vi "Test Selector Dialog.vi"(5 "Directory":path, 6 "Test Program":string, 7 "Test Names":string[](array[string]), 8 "error in":errorcluster, 9 "Test Available":bool[](array[boolean]), 10 "Limited Functional":bool[](array[boolean]), 11 "Test Selector":refnum<class "Test Selector.lvclass">) -> (0 "error out":errorcluster, 1 "Cancelled?":bool, 2 "Selected Tests":bool[](array[boolean]), 3 "Test Selector out":refnum<class "Test Selector.lvclass">, 4 "Limited Functional Flag":bool)   [LabVIEW 2019, in "Test Selector.lvlib" / "Test Selector.lvclass"]
uses:
  Test Selector.lvclass
  Test Selector.lvclass/Test Selector.ctl
  Accessors/Write Limited Functional Flag.vi
  Accessors/Read Limited Functional.vi
  Accessors/Read Selected Tests.vi
  Accessors/Read Test Available.vi
  Accessors/Write LstBox Refnum.vi
  Accessors/Write Test Names.vi
  Accessors/Write Limited Functional.vi
  Accessors/Write Test Available.vi
  Accessors/Write Test Program.vi
  Accessors/Write MissionLogo.vi
  Accessors/Write Directory.vi
  Accessors/Read Limited Functional Flag.vi
  Private/Fill Test Names.vi
  Private/Apply Symbols.vi
  Private/Process Selection.vi
panel:
  in  "Ltd Fnc":bool
  in  "Clear All":bool
  in  "Select All":bool
  in  "CANCEL":bool
  in  "DONE":bool
  in  "Selector":i32[](listbox)
  out "Dialog":string
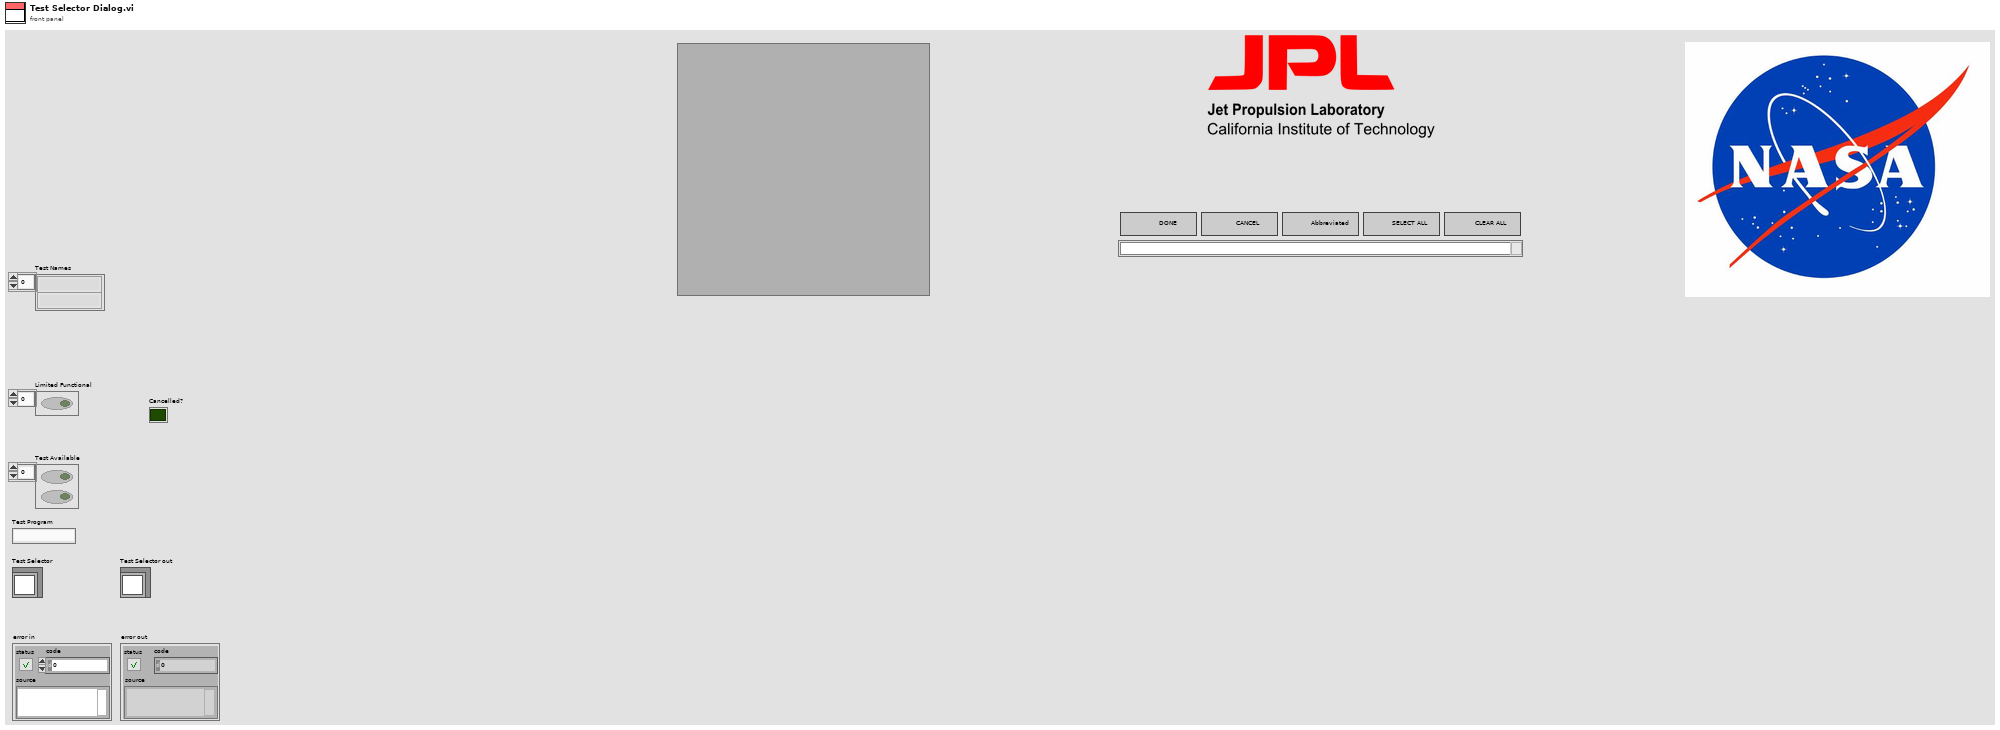
[diagram p1: front panel]
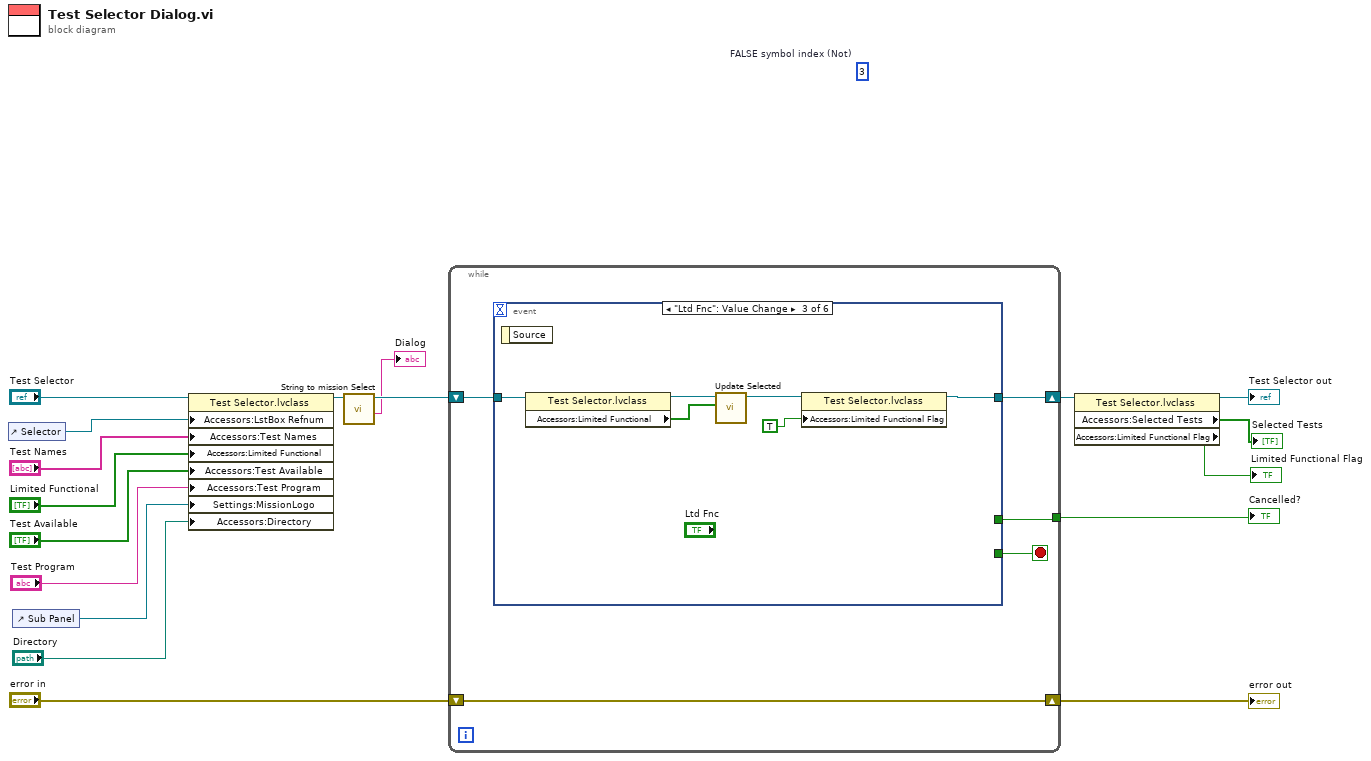
[diagram p0: block diagram]
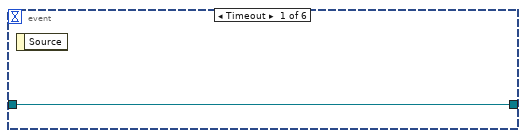
[diagram p2: hidden frame]
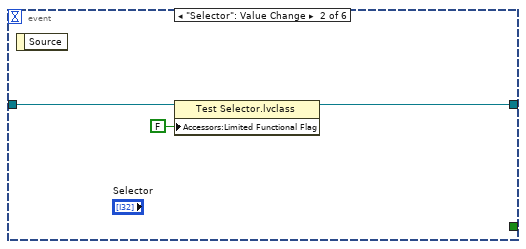
[diagram p3: hidden frame]
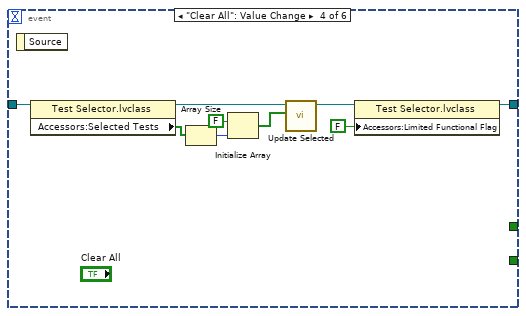
[diagram p4: hidden frame]
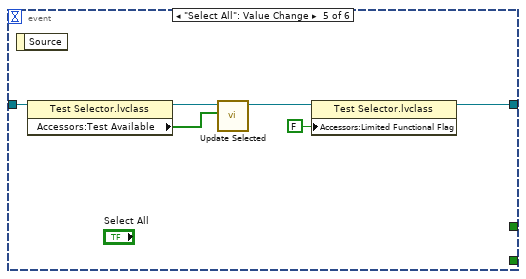
[diagram p5: hidden frame]
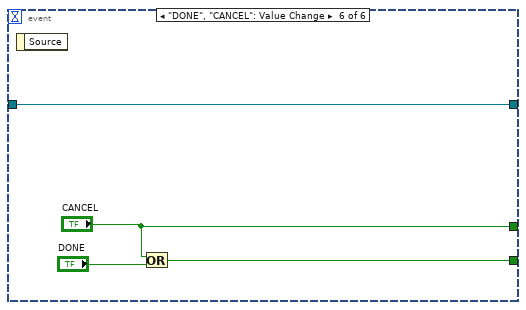
[diagram p6: hidden frame]
diagram:
  (unwired) 3  # FALSE symbol index (Not)
  n1 = control-ref of="Selector"() -> (w15:refnum<vi>)
  n2 = control-ref of="Sub Panel"() -> (w1:refnum<vi>)
  n3 = property class="Test Selector.lvclass"(reference="Test Selector", "Accessors:LstBox Refnum"=w15, "Accessors:Test Names"="Test Names", "Accessors:Limited Functional"="Limited Functional", "Accessors:Test Available"="Test Available", "Accessors:Test Program"="Test Program", "Settings:MissionLogo"=w1, "Accessors:Directory"="Directory") -> (reference out=w10:refnum<class "Test Selector.lvclass">)  [unwired: 1 in, 1 out]
  n4 = call "String to mission Select.vi"("Test Selector in"=w10) -> ("Test Dialog"=→"Dialog":string, "Test Selector out"=w9:refnum<class "Test Selector.lvclass">)  [unwired: 8 in, 1 out]
  n5 = while {
    shift-right: [w23] -> w18
    shift-left: "error in" -> [w23]
    shift-right: [w21] -> w8
    shift-left: w9 -> [w22]
    tunnel: [w19] -> w16
    stop <- w20 stop-if-true
    n6 = event shown="[2] \"Ltd Fnc\": Value Change" {
      selector: _ -> [_ _ _ _ _ _]
      dyn-events: _ -> [_ _ _ _ _ _]
      timeout: _ -> [_ _ _ _ _ _]
      tunnel: w22 -> [w24 w27 w33 w42 w48 w52]
      tunnel: [w24 w26 w29 w35 w44 w52] -> w21
      tunnel: [_ _ _ _ _ w50] -> w20
      tunnel: [_ _ _ _ _ "CANCEL"] -> w19
      event Timeout {
        n7 = event-data() -> ()  [unwired: 1 in, 1 out]
      }
      event "Selector": Value Change {
        n8 = event-data() -> ()  [unwired: 1 in, 1 out]
        n9 = property class="Test Selector.lvclass"(reference=w27, "Accessors:Limited Functional Flag"=FALSE ("Limited Functional Flag")) -> (reference out=w26:refnum<class "Test Selector.lvclass">)  [unwired: 1 in, 1 out]
      }
      event "Ltd Fnc": Value Change {
        n10 = event-data() -> ()  [unwired: 1 in, 1 out]
        n11 = property class="Test Selector.lvclass"(reference=w33) -> (reference out=w32:refnum<class "Test Selector.lvclass">, "Accessors:Limited Functional"=w31:bool[])  [unwired: 1 in, 1 out]
        n12 = call "Update Selected.vi"("Array"=w31, "Test Selector in"=w32) -> ("Test Selector out"=w30:refnum<class "Test Selector.lvclass">)  [unwired: 8 in, 1 out]
        n13 = property class="Test Selector.lvclass"(reference=w30, "Accessors:Limited Functional Flag"=TRUE) -> (reference out=w29:refnum<class "Test Selector.lvclass">)  [unwired: 1 in, 1 out]
      }
      event "Clear All": Value Change {
        n14 = event-data() -> ()  [unwired: 1 in, 1 out]
        n15 = property class="Test Selector.lvclass"(reference=w42) -> (reference out=w38:refnum<class "Test Selector.lvclass">, "Accessors:Selected Tests"=w40:bool[])  [unwired: 1 in, 1 out]
        n16 = Array Size(array=w40) -> (size(s)=w39:i32)
        n17 = Initialize Array(FALSE, w39) -> (w37:bool[])
        n18 = call "Update Selected.vi"("Array"=w37, "Test Selector in"=w38) -> ("Test Selector out"=w36:refnum<class "Test Selector.lvclass">)  [unwired: 8 in, 1 out]
        n19 = property class="Test Selector.lvclass"(reference=w36, "Accessors:Limited Functional Flag"=FALSE ("Limited Functional Flag")) -> (reference out=w35:refnum<class "Test Selector.lvclass">)  [unwired: 1 in, 1 out]
      }
      event "Select All": Value Change {
        n20 = event-data() -> ()  [unwired: 1 in, 1 out]
        n21 = property class="Test Selector.lvclass"(reference=w48) -> (reference out=w47:refnum<class "Test Selector.lvclass">, "Accessors:Test Available"=w45:bool[])  [unwired: 1 in, 1 out]
        n22 = call "Update Selected.vi"("Array"=w45, "Test Selector in"=w47) -> ("Test Selector out"=w46:refnum<class "Test Selector.lvclass">)  [unwired: 8 in, 1 out]
        n23 = property class="Test Selector.lvclass"(reference=w46, "Accessors:Limited Functional Flag"=FALSE ("Limited Functional Flag")) -> (reference out=w44:refnum<class "Test Selector.lvclass">)  [unwired: 1 in, 1 out]
      }
      event "DONE", "CANCEL": Value Change {
        n24 = event-data() -> ()  [unwired: 1 in, 1 out]
        n25 = Or(x="CANCEL", y="DONE") -> (x .or. y?=w50:bool)
      }
    }
  }
  "error out" <- w18
  "Cancelled?" <- w16
  n26 = property class="Test Selector.lvclass"(reference=w8) -> (reference out=→"Test Selector out":refnum<class "Test Selector.lvclass">, "Accessors:Selected Tests"=→"Selected Tests":bool[], "Accessors:Limited Functional Flag"=→"Limited Functional Flag":bool)  [unwired: 1 in, 1 out]
